vi "ma_Convert to One-sided Spectrum (complex).vi"(10 "spectrum type":enum16{"FFT spectrum", "cross spectrum"}(ring), 11 "two-sided spectrum (complex)":cdb[](array[numeric]) format="%0.2f") -> (2 "block size":dbl format="%0.2f", 3 "one-sided spectrum (complex)":cdb[](array[numeric]) format="%0.2f")   [LabVIEW 2020, in "NI_MAPro.lvlib"]
uses:
  NI_MAPro.lvlib
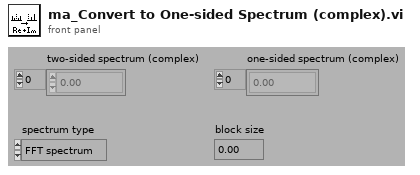
[diagram p1: front panel]
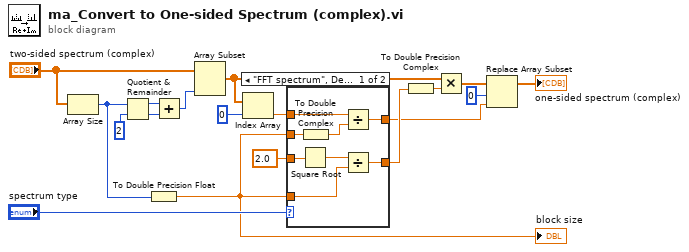
[diagram p0: block diagram]
diagram:
  n1 = Array Size(array="two-sided spectrum (complex)") -> (size(s)=w8:i32)
  n2 = Quotient & Remainder(x=w8, y=2) -> (x-y*floor(x/y)=w15:i32, floor(x/y)=w14:i32)
  n3 = To Double Precision Float(number=w8) -> (double precision float=w1:dbl)
  "block size" <- w1
  n4 = Add(x=w15, y=w14) -> (x+y=w13:i32)
  n5 = Array Subset(array="two-sided spectrum (complex)", length=w13) -> (w6:cdb[])  [unwired: 1 in]
  n6 = Index Array(array=w6, index=0) -> (element=w3:cdb)
  n7 = case shown="\"FFT spectrum\", Default" "spectrum type" {
    tunnel: 2.0 -> [w26 w28]
    tunnel: [w25 w28] -> w9
    tunnel: w1 -> [w22 _]
    tunnel: [w24 w27] -> w2
    tunnel: w3 -> [w23 w27]
    tunnel: w1 -> [w20 _]
    frame "FFT spectrum", Default {
      n8 = Square Root(x=w26) -> (sqrt(x)=w21:dbl)
      n9 = To Double Precision Complex(1:w20) -> (0:w19:cdb)
      n10 = Divide(x=w23, y=w19) -> (x/y=w24:cdb)
      n11 = Divide(x=w21, y=w22) -> (x/y=w25:dbl)
    }
    frame "cross spectrum" {
    }
  }
  n12 = To Double Precision Complex(1:w9) -> (0:w12:cdb)
  n13 = Multiply(x=w6, y=w12) -> (x*y=w10:cdb[])
  n14 = Replace Array Subset(array=w10, new element=w2, index=0 ("Index")) -> (→"one-sided spectrum (complex)":cdb[])
